vi "Create.vi"(8 "error in (no error)":errorcluster, 10 "Input":string) -> (0 "error out":errorcluster, 3 "Proto":refnum<class "Instruction.lvclass">)   [LabVIEW 2021, in "Instruction.lvclass"]
uses:
  Instruction.lvclass
  Instruction.lvclass/Instruction.ctl
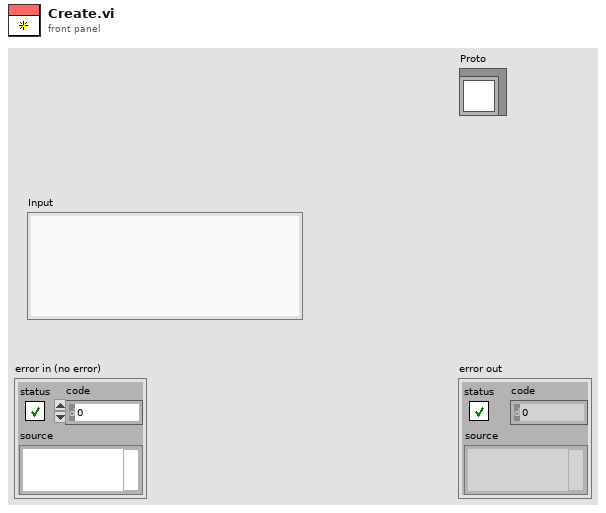
[diagram p1: front panel]
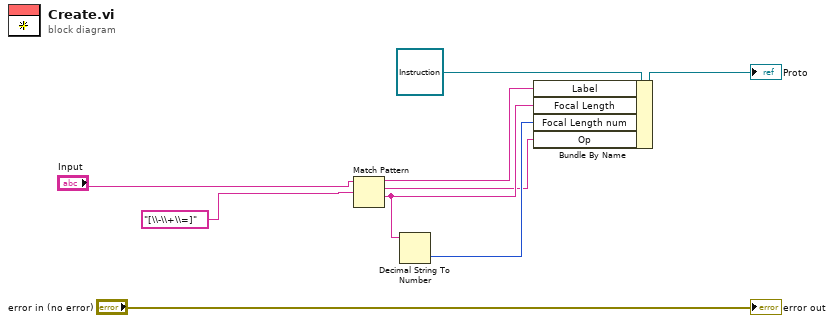
[diagram p0: block diagram]
diagram:
  n1 = Match Pattern(string="Input", regular expression="[\\-\\+\\=]" ("Delimiter regex")) -> (before substring=w1:string, match substring=w2:string, after substring=w3:string)  [unwired: 1 in, 1 out]
  n2 = Decimal String To Number(string=w3) -> (number=w4:i32)  [unwired: 2 in, 1 out]
  n3 = Bundle By Name(cluster=refnum<class "Instruction.lvclass"> refnum ("Proto"), "Label"=w1, "Focal Length"=w3, "Focal Length num"=w4, "Op"=w2) -> (→"Proto":refnum<class "Instruction.lvclass">)
  "error out" <- "error in (no error)"
